vi "SwerveDriveCalibrate.vi"() -> ()   [LabVIEW 2014]
uses:
  <vilib>/Platform/TimedLoop/XDataNode/timing_clust.ctl
  <vilib>/Platform/TimedLoop/XDataNode/nitl_modes.ctl
  <vilib>/Platform/TimedLoop/XDataNode/wakeup.ctl
  <vilib>/Rock Robotics/WPI/CAN/TalonSRX/WPI_CANTalonSRX_APIControlMode.ctl
  <vilib>/Rock Robotics/WPI/CAN/TalonSRX/WPI_CANTalonSRX_APIFeedbackSelect.ctl
  <vilib>/Rock Robotics/WPI/SafetyOutput/WPI_SafetyOutputConfigMenu.ctl
  <vilib>/Rock Robotics/WPI/MotorControl/WPI_MotorControlOpenCANTalonSRX.vi
  <vilib>/Platform/TimedLoop/XDataNode/XDataNode.xnode
  <vilib>/Rock Robotics/WPI/MotorControl/WPI_MotorControlType.ctl
  <vilib>/Rock Robotics/SystemInterfaces/Typedef/FPGA_TypedefDigitalModule.ctl
  <vilib>/Rock Robotics/SystemInterfaces/DIO/FPGA_DIOPWMChannel.ctl
  <vilib>/Rock Robotics/WPI/PWM/WPI_PWMDeadband.ctl
  <vilib>/Rock Robotics/WPI/CAN/Jaguar/SubVIs/WPI_CANJaguar_ControlMode.ctl
  <vilib>/Rock Robotics/WPI/PWM/WPI_PWMTransform_ConPane.ctl
  <vilib>/Rock Robotics/WPI/MotorControl/WPI_MotorControlDeviceRef.ctl
  <vilib>/Platform/TimedLoop/XDataNode/XDNodeRunTimeDep.lvlib
panel:
  in  "Ramp Rate":dbl=50.0
  out "Applied Throttle":dbl
  out "difference":dbl
  out "Analog In":dbl
  out "Encoder Position (-SRX)":dbl
  out "Sensor Position":dbl
  out "Quad velocities":dbl[](array[numeric])
  in  "Speed %VBus":dbl(slide) scale=-0.5..0.5
  out "Wheel Position":dbl(knob) scale=3.1416..-3.1416
  in  "Motor Controller":T1(ring)
  out "Waveform Chart":cluster{dbl, "motor output angle":dbl}(graph)
  in  "Enable":bool
  in  "Target Angle":dbl(knob) scale=3.1416..-3.1416
  in  "Offset":dbl
  in  "TPR":dbl=162.974661726
  in  "Set":bool
  in  "stop":bool
  out "error out":errorcluster
  in  "Steering PID":cluster{"P":dbl, "I":dbl, "D":dbl}={"P"=48.0, "I"=0.0, "D"=638.0}
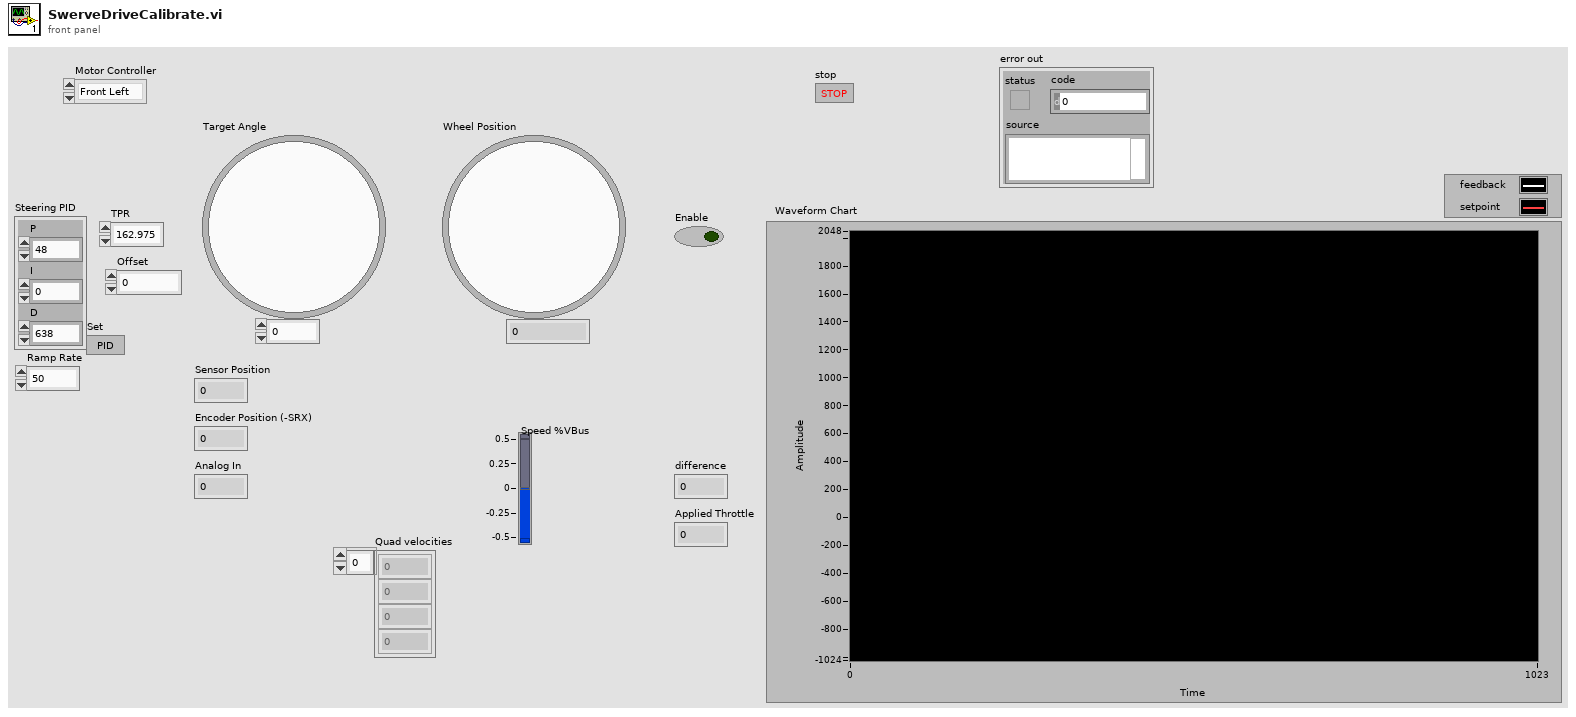
[diagram p1: front panel]
types:
  T1 = enum16{"Front Left", "Front Right", "Rear Left", "Rear Right"}
  T2 = typedef "WPI_MotorControlDeviceRef.ctl" = cluster{"DeviceStatus":errorcluster, "Type":T3, "PWM":cluster{"Controller":T4, "PWM Channel":T5, "DeadBand":T6}, "CAN":cluster{"Device Number":u8, "Control Mode":T7, "Semaphore":T8, "Max Vout":dbl, "TalonSRX Control Mode":T9}, "Invert":bool, "TransformRef":T10, "InvTransformRef":T10}
  T3 = typedef "WPI_MotorControlType.ctl" = enum16{"PWM", "CAN", "CANTalonSRX"}
  T4 = typedef "FPGA_TypedefDigitalModule.ctl" = enum16{"Controller 1"}
  T5 = typedef "FPGA_DIOPWMChannel.ctl" = enum8{"PWM 0", "PWM 1", "PWM 2", "PWM 3", "PWM 4", "PWM 5", "PWM 6", "PWM 7", "PWM 8", "PWM 9", "PWM MXP 0", "PWM MXP 1", "PWM MXP 2", "PWM MXP 3", "PWM MXP 4", "PWM MXP 5", "PWM MXP 6", "PWM MXP 7", "PWM MXP 8", "PWM MXP 9", "Invalid"}
  T6 = typedef "WPI_PWMDeadband.ctl" = cluster{"Name":string, "maxPositivePwm":i32, "minPositivePwm":i32, "centerPwm":i32, "maxNegativePwm":i32, "minNegativePwm":i32, "angularRange":u16}
  T7 = typedef "WPI_CANJaguar_ControlMode.ctl" = enum8{"Percent VBus", "Current", "Speed", "Position", "Voltage"}
  T8 = typedef "Semaphore RefNum" = refnum<k1>
  T9 = typedef "WPI_CANTalonSRX_APIControlMode.ctl" = enum8{"Percent VBus", "Speed", "Position", "Slave", "Unchanged / Invalid"}
  T10 = typedef "WPI_PWMTransform_ConPane.ctl" = refnum<vi>
  T11 = typedef "WPI_CANTalonSRX_APIFeedbackSelect.ctl" = enum16{"Digital Quadrature Encoder", "Analog Potentiometer", "Analog Encoder"}
  T12 = typedef "WPI_SafetyOutputConfigMenu.ctl" = enum16{"Enable", "Disable"}
  T13 = typedef "WPI_CANTalonSRX_GlobalStatus.ctl" = cluster{"Applied Throttle":dbl, "Module Enabled":bool, "CAN Error":errorcluster, "Closed Loop Error":dbl, "Forward Limit Switch Closed":bool, "Reverse Limit Switch Closed":bool, "Sensor Position":dbl, "Sensor Velocity":dbl, "Current":dbl, "Sticky Fault - Over Temp":bool, "Sticky Fault - Under Voltage":bool, "Sticky Fault - Forward Limit":bool, "Sticky Fault - Reverse Limit":bool, "Sticky Fault - Forward Soft Limit":bool, "Sticky Fault - Reverse Soft Limit":bool, "Brake is Enabled":bool, "Encoder Position":dbl, "Encoder Velocity":dbl, "Encoder Index Count":dbl, "Encoder A Pin State":bool, "Encoder B Pin State":bool, "Encoder Index Pin State":bool, "Analog In":dbl, "Analog In Velocity":dbl, "Temperature (C)":dbl, "Battery Voltage":dbl}
  T14 = typedef "XDNodeRunTimeDep.lvlib/timing_clust.ctl" = cluster{"Expected End [f-1]":u64, "Actual End [f-1]":u64, "Finished Late? [f-1]":bool, "Expected End [i-1]":u64, "Actual End [i-1]":u64, "Finished Late? [i-1]":bool, "Expected Start [i]":u64, "Actual Start [i]":u64, "Expected Start [f]":u64, "Actual Start [f]":u64, "Source Name":string, "Structure Name":string, "Period":i64, "Deadline":i64, "Offset":i64, "Start":i64, "Priority":i32, "Timeout":i32, "Mode":T15, "Wakeup Reason":T16, "Error":errorcluster, "Source Type":string, "Secondary Source Type":string, "Global End Time":u64, "Global Start Time":u64, "Frame Duration":u64, "Iteration Duration":u64, "Assigned CPU":i32, "I/O Scan Engine Mode":u32}
  T15 = typedef "XDNodeRunTimeDep.lvlib/nitl_modes.ctl" = enum32{"No Change", "Process missed periods, maintain original phase", "Discard missed periods, maintain original phase", "Process missed periods, ignore original phase", "Discard missed periods, ignore original phase"}
  T16 = typedef "XDNodeRunTimeDep.lvlib/wakeup.ctl" = enum32{"Normal", "Aborted", "Asynchronous wakeup", "Timing source error", "Timed loop error", "Timeout"}
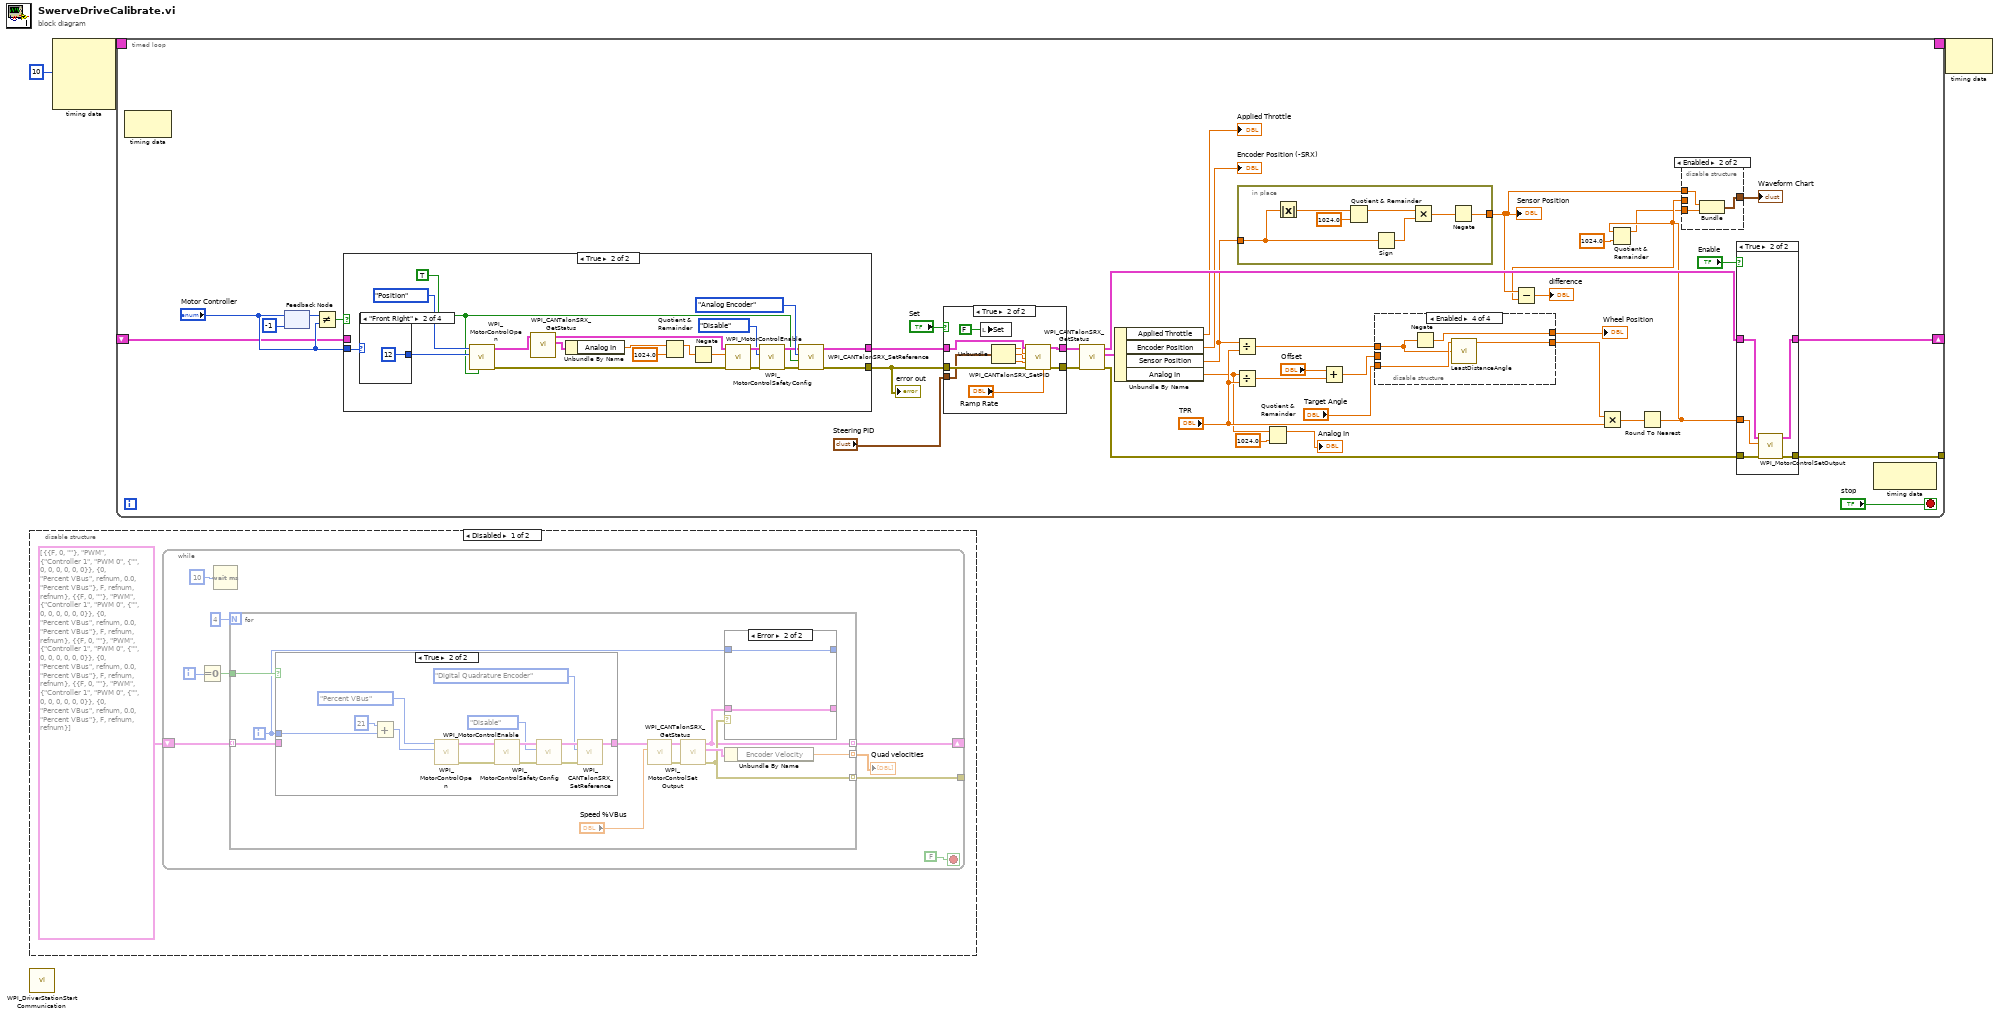
[diagram p0: block diagram]
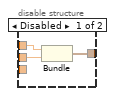
[diagram p5: hidden frame]
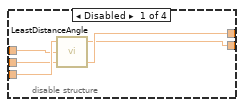
[diagram p6: hidden frame]
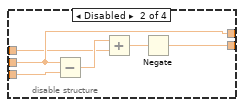
[diagram p7: hidden frame]
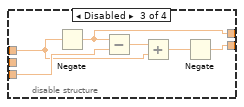
[diagram p8: hidden frame]
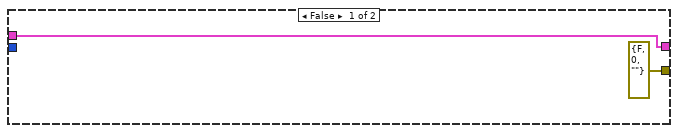
[diagram p9: hidden frame]
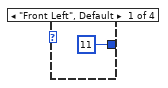
[diagram p10: hidden frame]
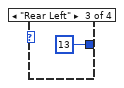
[diagram p11: hidden frame]
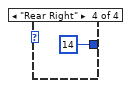
[diagram p12: hidden frame]
diagram:
  n1 = disable-structure shown="Disabled" {
    frame Disabled {
      n2 = while {
        shift-right: [w9] -> _
        shift-left: T2[] [{"DeviceStatus"={"status"=FALSE, "code"=0, "source"=""}, "Type"=enum."PWM", "PWM"={"Controller"=enum."Controller 1", "PWM Channel"=enum."PWM 0", "DeadBand"={"Name"="", "maxPositivePwm"=0, "minPositivePwm"=0, "centerPwm"=0, "maxNegativePwm"=0, "minNegativePwm"=0, "angularRange"=0}}, "CAN"={"Device Number"=0, "Control Mode"=enum."Percent VBus", "Semaphore"=refnum, "Max Vout"=0.0, "TalonSRX Control Mode"=enum."Percent VBus"}, "Invert"=FALSE, "TransformRef"=refnum, "InvTransformRef"=refnum}, {"DeviceStatus"={"status"=FALSE, "code"=0, "source"=""}, "Type"=enum."PWM", "PWM"={"Controller"=enum."Controller 1", "PWM Channel"=enum."PWM 0", "DeadBand"={"Name"="", "maxPositivePwm"=0, "minPositivePwm"=0, "centerPwm"=0, "maxNegativePwm"=0, "minNegativePwm"=0, "angularRange"=0}}, "CAN"={"Device Number"=0, "Control Mode"=enum."Percent VBus", "Semaphore"=refnum, "Max Vout"=0.0, "TalonSRX Control Mode"=enum."Percent VBus"}, "Invert"=FALSE, "TransformRef"=refnum, "InvTransformRef"=refnum}, {"DeviceStatus"={"status"=FALSE, "code"=0, "source"=""}, "Type"=enum."PWM", "PWM"={"Controller"=enum."Controller 1", "PWM Channel"=enum."PWM 0", "DeadBand"={"Name"="", "maxPositivePwm"=0, "minPositivePwm"=0, "centerPwm"=0, "maxNegativePwm"=0, "minNegativePwm"=0, "angularRange"=0}}, "CAN"={"Device Number"=0, "Control Mode"=enum."Percent VBus", "Semaphore"=refnum, "Max Vout"=0.0, "TalonSRX Control Mode"=enum."Percent VBus"}, "Invert"=FALSE, "TransformRef"=refnum, "InvTransformRef"=refnum}, {"DeviceStatus"={"status"=FALSE, "code"=0, "source"=""}, "Type"=enum."PWM", "PWM"={"Controller"=enum."Controller 1", "PWM Channel"=enum."PWM 0", "DeadBand"={"Name"="", "maxPositivePwm"=0, "minPositivePwm"=0, "centerPwm"=0, "maxNegativePwm"=0, "minNegativePwm"=0, "angularRange"=0}}, "CAN"={"Device Number"=0, "Control Mode"=enum."Percent VBus", "Semaphore"=refnum, "Max Vout"=0.0, "TalonSRX Control Mode"=enum."Percent VBus"}, "Invert"=FALSE, "TransformRef"=refnum, "InvTransformRef"=refnum}] -> [w8]
        tunnel: [w6] -> _
        i -> [w12]
        stop <- FALSE stop-if-true
        n3 = Equal To 0?(x=w12) -> (x = 0?=w10:bool)
        n4 = Wait (ms)(milliseconds to wait=u32 10) -> ()  [unwired: 1 out]
        n5 = for {
          N: 4 -> [_]
          tunnel: w10 -> [w24]
          tunnel: [w14] -> w9 mode=indexing
          tunnel: w8 -> [w23] mode=indexing
          tunnel: [w16] -> w6 mode=indexing
          tunnel: [w17] -> w5 mode=indexing
          i -> [w15]
          n6 = case shown="True" w24 {
            tunnel: [w29 w31] -> w22
            tunnel: w23 -> [w29 _]
            tunnel: w15 -> [_ w35]
            frame False {
            }
            frame True {
              n7 = Add(x=21, y=w35) -> (x+y=w34:i32)
              n8 = call-poly <vilib>:"WPI_MotorControlOpen.vi"("Device Number"=w34, "Control Mode"=WPI_CANTalonSRX_APIControlMode."Percent VBus") -> ("error out"=w41:errorcluster, "MotorControlDeviceRef"=w40:T2)  [unwired: 8 in]
              n9 = call <vilib>:"WPI_MotorControlEnable.vi"("error in (no error)"=w41, "CAN Jaguar Ref"=w40) -> ("error out"=w38:errorcluster, "CAN Jaguar Ref Out"=w39:T2)  [unwired: 8 in]
              n10 = call <vilib>:"WPI_MotorControlSafetyConfig.vi"("error in (no error)"=w38, "mode"=WPI_SafetyOutputConfigMenu."Disable", "MotorControlDevRef"=w39) -> ("error out"=w32:errorcluster, "MotorControlDevRef"=w33:T2)  [unwired: 7 in]
              n11 = call <vilib>:"WPI_CANTalonSRX_SetReference.vi"("error in (no error)"=w32, "Feedback Reference"=WPI_CANTalonSRX_APIFeedbackSelect."Digital Quadrature Encoder", "CAN Talon SRX Ref"=w33) -> ("CAN Talon SRX Ref Out"=w31:T2)  [unwired: 7 in, 1 out]
            }
          }
          n12 = call <vilib>:"WPI_MotorControlSetOutput.vi"("Output"="Speed %VBus", "MotorControlDevRef"=w22) -> ("error out"=w20:errorcluster, "MotorControlDevRef"=w19:T2)  [unwired: 7 in, 1 out]
          n13 = call <vilib>:"WPI_CANTalonSRX_GetStatus.vi"("error in (no error)"=w20, "CAN Talon SRX Ref"=w19) -> ("error out"=w16:errorcluster, "Talon SRX Status"=w18:T13, "CAN Talon SRX Ref Out"=w14:T2)  [unwired: 7 in]
          n14 = case shown="Error" w16 {
            tunnel: [w26 w27] -> _
            tunnel: w15 -> [w26 w27]
            tunnel: [w25 w28] -> _
            tunnel: w14 -> [w25 w28]
            frame No Error {
            }
            frame Error {
            }
          }
          n15 = Unbundle By Name(w18) -> ("Encoder Velocity"=w17:dbl)
        }
        "Quad velocities" <- w5
      }
    }
    frame Enabled {
    }
  }
  n16 = call <vilib>:"WPI_DriverStationStart Communication.vi"() -> ()  [unwired: 12 in]
  n17 = node-c288(i64 10 ("Period")) -> (w3:T14)  [unwired: 3 in]
  n18 = timed-loop {
    timing: w3 -> [_]
    timing-out: [_] -> w2
    shift-right: [w70] -> _
    shift-left: _ -> [w62]
    tunnel: [w57] -> _
    stop <- "stop" stop-if-true
    n19 = node-c288() -> ()  [unwired: 1 in, 1 out]
    n20 = feedback-in #1("Motor Controller") -> ()
    n21 = feedback #1(-1) -> (w67:i32)
    n22 = Not Equal?(x=w67, y="Motor Controller") -> (x != y?=w64:bool)
    n23 = case shown="True" w64 {
      tunnel: "Motor Controller" -> [_ w132]
      tunnel: [w117 w131] -> w69
      tunnel: [errorcluster {"status"=FALSE, "code"=0, "source"=""} ("error out") w130] -> w68
      tunnel: w62 -> [w117 _]
      frame False {
      }
      frame True {
        w124 = TRUE ("Invert")
        n24 = case shown="\"Front Right\"" w132 {
          tunnel: [11 12 13 14] -> w134
          frame "Front Left", Default {
          }
          frame "Front Right" {
          }
          frame "Rear Left" {
          }
          frame "Rear Right" {
          }
        }
        n25 = call-poly <vilib>:"WPI_MotorControlOpen.vi"("Invert"=w124, "Device Number"=w134, "Control Mode"=WPI_CANTalonSRX_APIControlMode."Position") -> ("error out"=w136:errorcluster, "MotorControlDeviceRef"=w135:T2)  [unwired: 7 in]
        n26 = call <vilib>:"WPI_CANTalonSRX_GetStatus.vi"("CAN Talon SRX Ref"=w135) -> ("Talon SRX Status"=w122:T13, "CAN Talon SRX Ref Out"=w123:T2)  [unwired: 8 in, 1 out]
        n27 = Unbundle By Name(w122) -> ("Analog In"=w120:dbl)
        n28 = Quotient & Remainder(x=w120, y=1024.0) -> (x-y*floor(x/y)=w119:dbl)  [unwired: 1 out]
        n29 = Negate(x=w119) -> (-x=w118:dbl)
        n30 = call <vilib>:"WPI_MotorControlEnable.vi"("error in (no error)"=w136, "Encoder Initial Position"=w118, "CAN Jaguar Ref"=w123) -> ("error out"=w128:errorcluster, "CAN Jaguar Ref Out"=w129:T2)  [unwired: 7 in]
        n31 = call <vilib>:"WPI_MotorControlSafetyConfig.vi"("error in (no error)"=w128, "mode"=WPI_SafetyOutputConfigMenu."Disable", "MotorControlDevRef"=w129) -> ("error out"=w127:errorcluster, "MotorControlDevRef"=w126:T2)  [unwired: 7 in]
        n32 = call <vilib>:"WPI_CANTalonSRX_SetReference.vi"("error in (no error)"=w127, "Reverse Feedback Sensor"=w124, "Feedback Reference"=WPI_CANTalonSRX_APIFeedbackSelect."Analog Encoder", "CAN Talon SRX Ref"=w126) -> ("error out"=w130:errorcluster, "CAN Talon SRX Ref Out"=w131:T2)  [unwired: 6 in]
      }
    }
    "error out" <- w68
    n33 = case shown="True" "Set" {
      tunnel: w69 -> [w150 w159]
      tunnel: w68 -> [w149 w158]
      tunnel: [w149 w157] -> w79
      tunnel: [w150 w156] -> w78
      tunnel: "Steering PID" -> [_ w152]
      frame False {
      }
      frame True {
        n34 = local write "Set"(FALSE) -> ()
        n35 = Unbundle(w152) -> ("P"=w155:dbl, "I"=w154:dbl, "D"=w153:dbl)
        n36 = call <vilib>:"WPI_CANTalonSRX_SetPID.vi"("CAN Talon SRX Ref"=w159, "P"=w155, "I"=w154, "D"=w153, "error in (no error)"=w158, "Ramp Rate"="Ramp Rate") -> ("CAN Talon SRX Ref Out"=w156:T2, "error out"=w157:errorcluster)  [unwired: 8 in]
      }
    }
    n37 = call <vilib>:"WPI_CANTalonSRX_GetStatus.vi"("error in (no error)"=w79, "CAN Talon SRX Ref"=w78) -> ("error out"=w75:errorcluster, "Talon SRX Status"=w80:T13, "CAN Talon SRX Ref Out"=w74:T2)  [unwired: 7 in]
    n38 = Unbundle By Name(w80) -> ("Applied Throttle"=→"Applied Throttle":dbl, "Encoder Position"=→"Encoder Position (-SRX)":dbl, "Sensor Position"=w47:dbl, "Analog In"=w48:dbl)
    n39 = Divide(x=w47, y="TPR") -> (x/y=w54:dbl)
    n40 = Divide(x=w48, y="TPR") -> (x/y=w61:dbl)
    n41 = in-place {
      in-place-border: [w88] -> w46
      in-place-border: w47 -> [w92]
      n42 = Absolute Value(x=w92) -> (abs(x)=w93:dbl)
      n43 = Quotient & Remainder(x=w93, y=1024.0) -> (x-y*floor(x/y)=w91:dbl)  [unwired: 1 out]
      n44 = Sign(1:w92) -> (0:w90:dbl)
      n45 = Multiply(x=w91, y=w90) -> (x*y=w89:dbl)
      n46 = Negate(x=w89) -> (-x=w88:dbl)
    }
    "Sensor Position" <- w46
    n47 = Quotient & Remainder(x=w48, y=1024.0) -> (x-y*floor(x/y)=→"Analog In":dbl)  [unwired: 1 out]
    n48 = Add(x="Offset", y=w61) -> (x+y=w59:dbl)
    n49 = disable-structure shown="Enabled" {
      disable-tunnel: [w95 w100 w108 w113] -> w76
      disable-tunnel: "Target Angle" -> [w99 w105 w111 w115]
      disable-tunnel: w59 -> [w98 w103 _ _]
      disable-tunnel: [w97 w103 w107 w112] -> w58
      disable-tunnel: w54 -> [w96 w101 w106 w114]
      frame Disabled {
        n50 = call "LeastDistanceAngle.vi"(3:w98, "Sensor position"=w96, "target angle (between pi and -pi)"=w99) -> ("current angle (between pi and -pi)"=w97:dbl, "motor output angle"=w95:dbl)  [unwired: 1 out]
      }
      frame Disabled {
        n51 = Subtract(x=w103, y=w105) -> (x-y=w102:dbl)
        n52 = Add(x=w102, y=w101) -> (x+y=w104:dbl)
        n53 = Negate(x=w104) -> (-x=w100:dbl)
      }
      frame Disabled {
        n54 = Negate(x=w106) -> (-x=w107:dbl)
        n55 = Subtract(x=w107, y=w111) -> (x-y=w109:dbl)
        n56 = Add(x=w109, y=w106) -> (x+y=w110:dbl)
        n57 = Negate(x=w110) -> (-x=w108:dbl)
      }
      frame Enabled {
        n58 = Negate(x=w114) -> (-x=w112:dbl)
        n59 = call "LeastDistanceAngle.vi"("Sensor position"=w114, "target angle (between pi and -pi)"=w115) -> ("motor output angle"=w113:dbl)  [unwired: 1 in, 2 out]
      }
    }
    "Wheel Position" <- w58
    n60 = Multiply(x=w76, y="TPR") -> (x*y=w51:dbl)
    n61 = Round To Nearest(number=w51) -> (nearest integer value=w44:dbl)
    n62 = Subtract(x=w46, y=w44) -> (x-y=→"difference":dbl)
    n63 = Quotient & Remainder(x=w44, y=1024.0) -> (x-y*floor(x/y)=w43:dbl)  [unwired: 1 out]
    n64 = disable-structure shown="Enabled" {
      disable-tunnel: [w84 w87] -> w72
      disable-tunnel: w46 -> [w83 w85]
      disable-tunnel: w44 -> [w82 _]
      disable-tunnel: w43 -> [_ w86]
      frame Disabled {
        n65 = Bundle(w83, w82) -> (w84:cluster{dbl, dbl})  [unwired: 1 in]
      }
      frame Enabled {
        n66 = Bundle(w85, w86) -> (w87:cluster{dbl, dbl})  [unwired: 1 in]
      }
    }
    "Waveform Chart" <- w72
    n67 = case shown="True" "Enable" {
      tunnel: w75 -> [w143 w148]
      tunnel: [w143 w147] -> w57
      tunnel: w74 -> [w142 w146]
      tunnel: [w142 w145] -> w70
      tunnel: w44 -> [_ w144]
      frame False {
      }
      frame True {
        n68 = call <vilib>:"WPI_MotorControlSetOutput.vi"("error in (no error)"=w148, "Output"=w144, "MotorControlDevRef"=w146) -> ("error out"=w147:errorcluster, "MotorControlDevRef"=w145:T2)  [unwired: 6 in, 1 out]
      }
    }
    n69 = node-c288() -> ()  [unwired: 1 in, 1 out]
  }
  n70 = node-c288(w2) -> ()  [unwired: 1 out]
